vi "Apply Config.vi"(8 "ErrorIn":errorcluster, 10 "Name":string, 11 "TopModuleIn":refnum<class "Logger.lvclass">) -> (0 "ErrorOut":errorcluster, 3 "TopModuleOut":refnum<class "Logger.lvclass">)   [LabVIEW 2019, in "Logger.lvclass"]
uses:
  Logger.lvclass
  IConfig/IConfig.lvclass
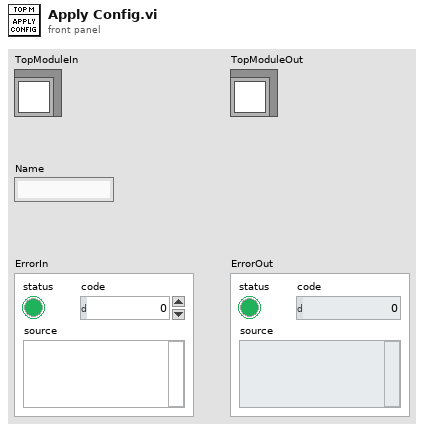
[diagram p1: front panel]
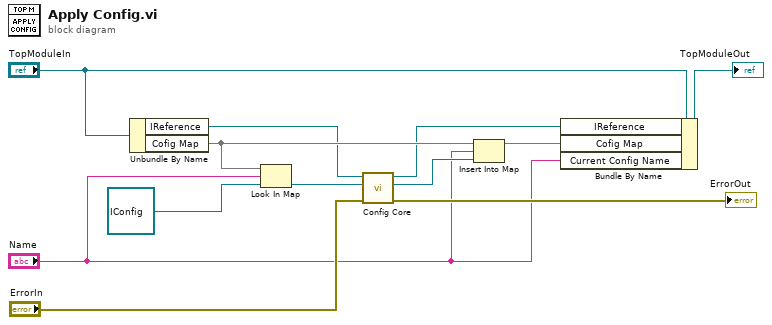
[diagram p0: block diagram]
diagram:
  n1 = Unbundle By Name("TopModuleIn") -> ("IReference"=w5:refnum<class "IReference.lvclass">, "Cofig Map"=w7:map{string, refnum<class "IConfig.lvclass">})
  n2 = Look In Map(map=w7, key="Name", default value=refnum<class "IConfig.lvclass"> refnum ("IConfig.lvclass")) -> (value=w6:refnum<class "IConfig.lvclass">)  [unwired: 1 out]
  n3 = call-dynamic "Config Core.vi"("Error In"="ErrorIn", "IConfigIn"=w6, "HardwareIn"=w5) -> ("Error Out"=→"ErrorOut":errorcluster, "IConfigOut"=w3:refnum<class "IConfig.lvclass">, "HardwareOut"=w4:refnum<class "IReference.lvclass">)  [unwired: 6 in]
  n4 = Insert Into Map(map in=w7, key="Name", value=w3) -> (map out=w2:map{string, refnum<class "IConfig.lvclass">})  [unwired: 2 out]
  n5 = Bundle By Name(cluster="TopModuleIn", "IReference"=w4, "Cofig Map"=w2, "Current Config Name"="Name") -> (→"TopModuleOut":refnum<class "Logger.lvclass">)
